vi "Build Evaluation String.vi"(6 "VI Path":path, 7 "Assert Scripting Configuration":T1={"Assert Name"="", "Comment"="", "Numeric Operation"="", "Type"=enum."Double Float", "String Operation"="", "DBL Comparison Value 1"=0.0, "DBL Comparison Value 2"=0.0, "I32 Comparison Value 1"=0, "I32 Comparison Value 2"=0, "Creator"="", "Creation Timestamp"=timestamp(0 s since 1904-01-01), "String Comparison Value"="", "Description"="", "Default Failure Action"=enum."None", "Boolean Comparison Value"=FALSE}, 8 "error in (no error)":errorcluster) -> (0 "error out":errorcluster, 2 "Evaluation String":string)   [LabVIEW 2016]
doc: "Builds up an evaluation string based on the input parameters specified and applies it to the new assert test vi."
uses:
  Assert Scripting Configuration.ctl
  <vilib>/Utility/Data Type/Type Definitions/Data Type.ctl
  <vilib>/Utility/Data Type/NI_Data Type.lvlib
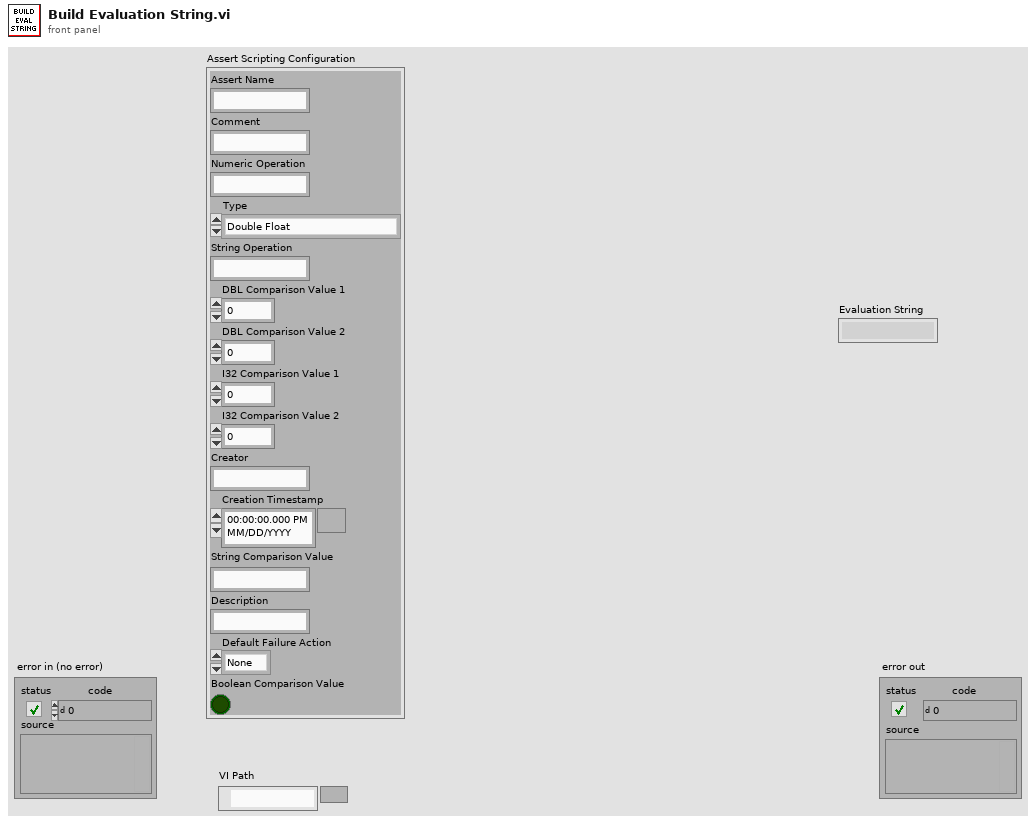
[diagram p1: front panel]
types:
  T1 = typedef "Assert Scripting Configuration.ctl" = cluster{"Assert Name":string, "Comment":string, "Numeric Operation":string, "Type":T2, "String Operation":string, "DBL Comparison Value 1":dbl, "DBL Comparison Value 2":dbl, "I32 Comparison Value 1":i32, "I32 Comparison Value 2":i32, "Creator":string, "Creation Timestamp":timestamp, "String Comparison Value":string, "Description":string, "Default Failure Action":enum16{"None", "Log To File", "Pause Execution", "Abort Execution"}, "Boolean Comparison Value":bool}
  T2 = typedef "NI_Data Type.lvlib/Data Type.ctl" = enum8{"Invalid Type", "Void", "I8", "I16", "I32", "I64", "U8", "U16", "U32", "U64", "Single Float", "Double Float", "Extended Float", "Single Complex", "Double Complex", "Extended Complex", "Enum U8", "Enum U16", "Enum U32", "Enum U64", "Single Float With Unit", "Double Float With Unit", "Extended Float With Unit", "Single Complex with Unit", "Double Complex with Unit", "Extended Complex with Unit", "Boolean", "String", "Path", "Picture", "Tag", "Array", "Cluster", "Variant", "LV Variant", "Waveform", "Timestamp", "Digital Waveform", "Digital Data", "ExpressData", "Refnum", "External Data", "VI", "Poly VI", "LabVIEW Class Instance", "Fixed Point"}
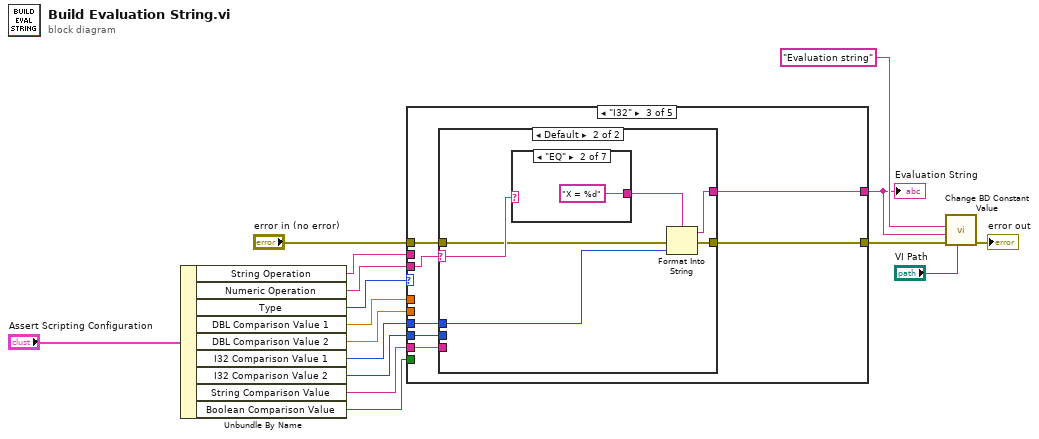
[diagram p0: block diagram]
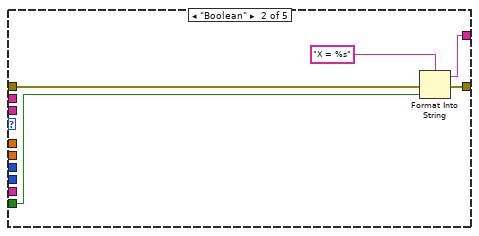
[diagram p3: hidden frame]
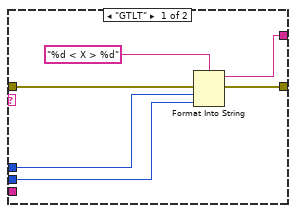
[diagram p4: hidden frame]
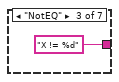
[diagram p6: hidden frame]
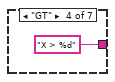
[diagram p7: hidden frame]
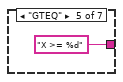
[diagram p8: hidden frame]
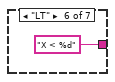
[diagram p9: hidden frame]
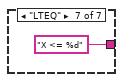
[diagram p10: hidden frame]
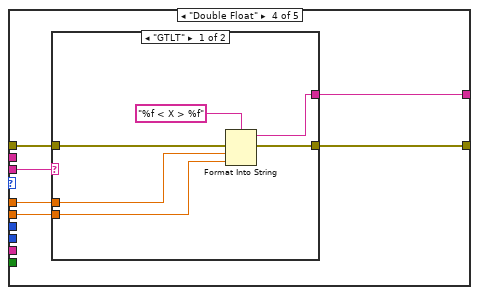
[diagram p11: hidden frame]
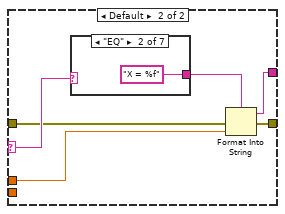
[diagram p12: hidden frame]
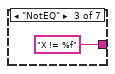
[diagram p14: hidden frame]
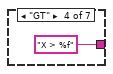
[diagram p15: hidden frame]
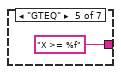
[diagram p16: hidden frame]
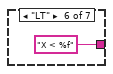
[diagram p17: hidden frame]
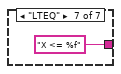
[diagram p18: hidden frame]
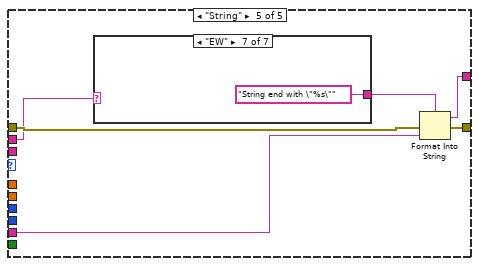
[diagram p19: hidden frame]
diagram:
  n1 = Unbundle By Name("Assert Scripting Configuration") -> ("String Operation"=w12:string, "Numeric Operation"=w13:string, "Type"=w14:T2, "DBL Comparison Value 1"=w8:dbl, "DBL Comparison Value 2"=w7:dbl, "I32 Comparison Value 1"=w11:i32, "I32 Comparison Value 2"=w10:i32, "String Comparison Value"=w6:string, "Boolean Comparison Value"=w1:bool)
  n2 = case shown="\"I32\"" w14 {
    tunnel: w13 -> [_ _ w29 w53 _]
    tunnel: w12 -> [_ _ _ _ w74]
    tunnel: w11 -> [_ _ w28 _ _]
    tunnel: w10 -> [_ _ w27 _ _]
    tunnel: [_ w20 w26 w52 w72] -> w5
    tunnel: "error in (no error)" -> [w17 w19 w25 w51 w77]
    tunnel: [w17 w18 w24 w50 w76] -> w4
    tunnel: w8 -> [_ _ _ w49 _]
    tunnel: w7 -> [_ _ _ w48 _]
    tunnel: w6 -> [_ _ w23 _ w75]
    tunnel: w1 -> [_ w22 _ _ _]
    frame Default {
    }
    frame "Boolean" {
      n3 = Format Into String(format string="X = %s", error in=w19, w22) -> (resulting string=w20:string, error out=w18:errorcluster)  [unwired: 1 in]
    }
    frame "I32" {
      n4 = case shown="Default" w29 {
        selector: w29 -> [_ w41]
        tunnel: w28 -> [w35 w39]
        tunnel: w27 -> [w34 _]
        tunnel: [w32 w38] -> w26
        tunnel: w25 -> [w31 w37]
        tunnel: [w30 w36] -> w24
        tunnel: w23 -> [_ _]
        frame "GTLT" {
          n5 = Format Into String(format string="%d < X > %d", error in=w31, w35, w34) -> (resulting string=w32:string, error out=w30:errorcluster)  [unwired: 1 in]
        }
        frame Default {
          n6 = case shown="\"EQ\"" w41 {
            tunnel: [_ "X = %d" "X != %d" "X > %d" "X >= %d" "X < %d" "X <= %d"] -> w40
            frame Default {
            }
            frame "EQ" {
            }
            frame "NotEQ" {
            }
            frame "GT" {
            }
            frame "GTEQ" {
            }
            frame "LT" {
            }
            frame "LTEQ" {
            }
          }
          n7 = Format Into String(format string=w40, error in=w37, w39) -> (resulting string=w38:string, error out=w36:errorcluster)  [unwired: 1 in]
        }
      }
    }
    frame "Double Float" {
      n8 = case shown="\"GTLT\"" w53 {
        selector: w53 -> [_ w65]
        tunnel: w49 -> [w59 w63]
        tunnel: w48 -> [w58 _]
        tunnel: [w56 w62] -> w52
        tunnel: w51 -> [w55 w61]
        tunnel: [w54 w60] -> w50
        frame "GTLT" {
          n9 = Format Into String(format string="%f < X > %f", error in=w55, w59, w58) -> (resulting string=w56:string, error out=w54:errorcluster)  [unwired: 1 in]
        }
        frame Default {
          n10 = case shown="\"EQ\"" w65 {
            tunnel: [_ "X = %f" "X != %f" "X > %f" "X >= %f" "X < %f" "X <= %f"] -> w64
            frame Default {
            }
            frame "EQ" {
            }
            frame "NotEQ" {
            }
            frame "GT" {
            }
            frame "GTEQ" {
            }
            frame "LT" {
            }
            frame "LTEQ" {
            }
          }
          n11 = Format Into String(format string=w64, error in=w61, w63) -> (resulting string=w62:string, error out=w60:errorcluster)  [unwired: 1 in]
        }
      }
    }
    frame "String" {
      n12 = case shown="\"EW\"" w74 {
        tunnel: [_ "String = \"%s\"" "String != \"%s\"" "String should contain \"%s\"" "String should not contain \"%s\"" "String start with \"%s\"" "String end with \"%s\""] -> w73
        frame Default {
        }
        frame "EQ" {
        }
        frame "NotEQ" {
        }
        frame "Contains" {
        }
        frame "NotContain" {
        }
        frame "SW" {
        }
        frame "EW" {
        }
      }
      n13 = Format Into String(format string=w73, error in=w77, w75) -> (resulting string=w72:string, error out=w76:errorcluster)  [unwired: 1 in]
    }
  }
  "Evaluation String" <- w5
  n14 = call "Change BD Constant Value.vi"("Assert VI Path"="VI Path", "error in (no error)"=w4, "Data Value"=w5, "Constant Name"="Evaluation string") -> ("error out"=→"error out":errorcluster)  [unwired: 7 in]
